vi "Read Measurement (Occupied Bandwidth).vi"(8 "error in (no error)":errorcluster, 9 "Maximum Time (20000 ms)":i32=20000, 11 "VISA resource name":refnum<visa-resource-name>) -> (0 "error out":errorcluster, 1 "Occupied Bandwidth (Hz)":dbl format="%#.6g", 2 "Transmit Frequency Error (Hz)":dbl format="%#.6g", 3 "VISA resource name out":refnum<visa-resource-name>, 5 "x dB Bandwidth (Hz)":dbl format="%#.6g")   [LabVIEW 2014, in "Agilent ESA PSA Series.lvlib"]
doc: "Stops the present measurement and sets up the instrument for the a occupied bandwidth measurements.\n\nAfter the data are valid, the scalar result is returned for the specified measurement. These are the settings and units that conform to the measurement specific standard.\n\n- Stops the current measurement and does not reset the measurement to the factory defaults.\n\n- Initiates the measurement and puts valid data into the output buffer. If a measurement other than the current one is specified, the instrument will switch to that measurement before it initiates the measurement and returns results.\n\n- Blocks other SCPI communication, waiting until the measurement is complete before returning results."
uses:
  Agilent ESA PSA Series.lvlib
  Fetch Measurement (Occupied Bandwidth).vi
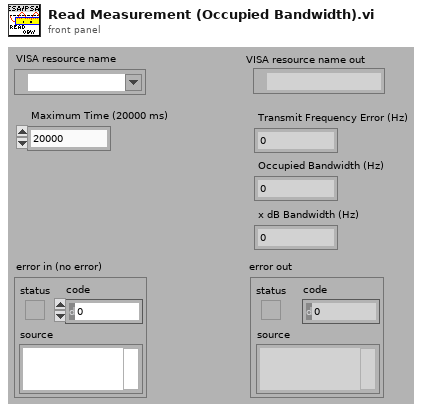
[diagram p1: front panel]
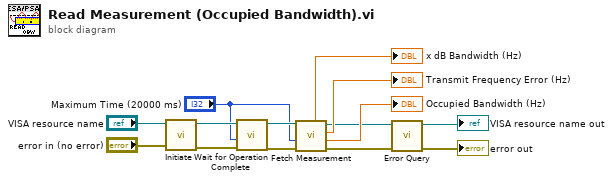
[diagram p0: block diagram]
diagram:
  n1 = call "Initiate.vi"("error in (no error)"="error in (no error)", "VISA resource name"="VISA resource name") -> ("error out"=w11:errorcluster, "VISA resource name out"=w12:refnum<visa-resource-name>)  [unwired: 8 in]
  n2 = call "Wait for Operation Complete.vi"("error in (no error)"=w11, "Maximum Time (10000ms)"="Maximum Time (20000 ms)", "VISA resource name"=w12) -> ("error out"=w9:errorcluster, "VISA resource name out"=w10:refnum<visa-resource-name>)  [unwired: 7 in]
  n3 = call-poly "Fetch Measurement.vi"("error in (no error)"=w9, "Timeout (20000 ms)"="Maximum Time (20000 ms)", "VISA resource name"=w10) -> ("error out"=w4:errorcluster, "Occupied Bandwidth (Hz)"=→"Occupied Bandwidth (Hz)":dbl, "Transmit Frequency Error (Hz)"=→"Transmit Frequency Error (Hz)":dbl, "VISA resource name out"=w5:refnum<visa-resource-name>, "x dB Bandwidth (Hz)"=→"x dB Bandwidth (Hz)":dbl)  [unwired: 4 in]
  n4 = call "Error Query.vi"("error in (no error)"=w4, "VISA resource name"=w5) -> ("error out"=→"error out":errorcluster, "VISA resource name out"=→"VISA resource name out":refnum<visa-resource-name>)  [unwired: 6 in, 2 out]
